vi "Kaelus PIM Add Model with Serial Numbers to Tree.vi"(4 "Instrument Index":i32, 6 "Model Serial Numbers":string[](array[string]), 8 "error in (no error)":errorcluster, 9 "Model Descriptive Columns":string[](array[string]), 10 "Model Name":string="Model", 11 "Tree Control Reference":refnum<vi>) -> (0 "error out":errorcluster)   [LabVIEW 2011]
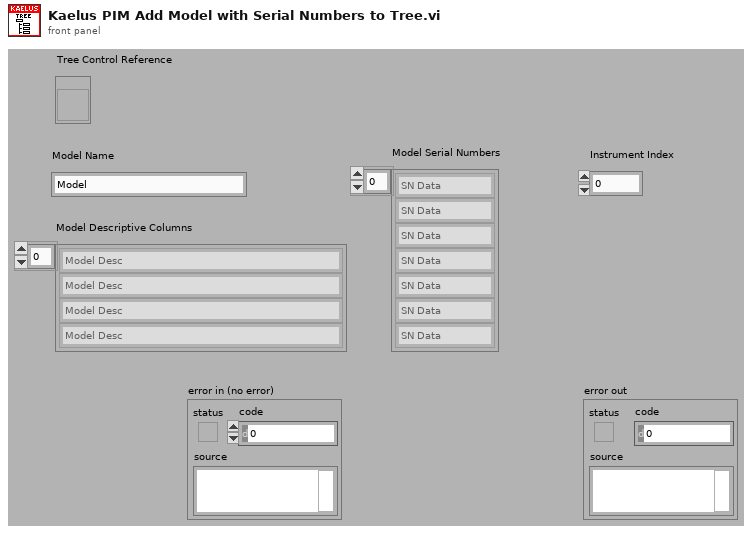
[diagram p1: front panel]
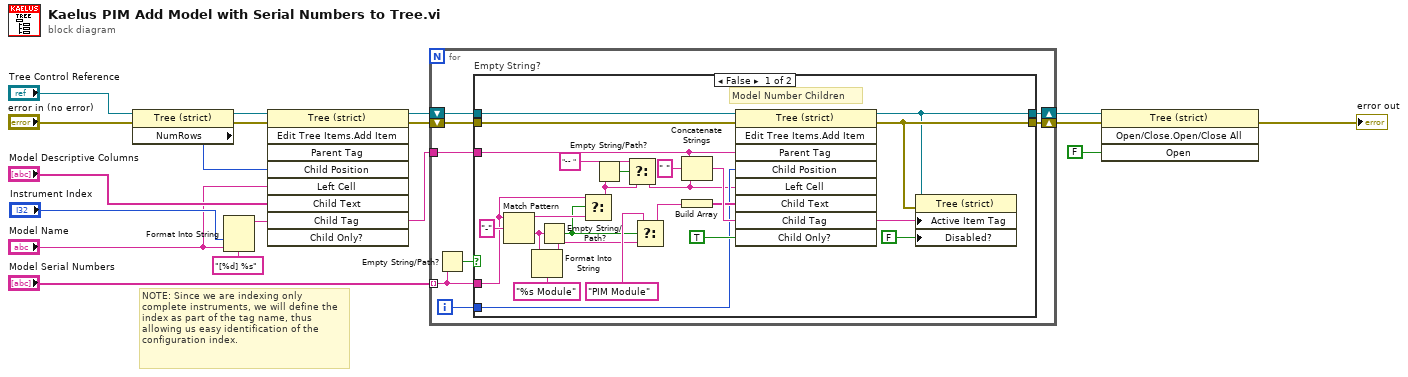
[diagram p0: block diagram]
diagram:
  # "NOTE: Since we are indexing only complete instruments, we will define the index as part of the tag name, thus allowing us easy identification of the configuration index."
  n1 = property class="Tree (strict)"(reference="Tree Control Reference", error in="error in (no error)") -> (reference out=w3:refnum<vi>, error out=w2:errorcluster, "NumRows"=w1:u32)
  n2 = Format Into String(format string="[%d] %s", "Instrument Index", "Model Name") -> (resulting string=w17:string)  [unwired: 2 in, 1 out]
  n3 = invoke class="Tree (strict)" method="Edit Tree Items.Add Item"(reference=w3, error in=w2, "Child Position"=w1, "Left Cell"="Model Name", "Child Text"="Model Descriptive Columns", "Child Tag"=w17) -> (reference out=w16:refnum<vi>, error out=w13:errorcluster)  [unwired: 3 in, 7 out]
  n4 = for {
    tunnel: w17 -> [w21]
    tunnel: "Model Serial Numbers" -> [w18] mode=indexing
    shift-right: [w23] -> w7
    shift-left: w13 -> [w24]
    shift-right: [w22] -> w8
    shift-left: w16 -> [w25]
    i -> [w20]
    n5 = Empty String/Path?(string/path=w18) -> (empty?=w19:bool)
    n6 = case "Empty String?" shown="False" w19 {
      tunnel: w25 -> [w32 w51]
      tunnel: w24 -> [w33 w50]
      tunnel: [w27 w50] -> w23
      tunnel: [w26 w51] -> w22
      tunnel: w18 -> [w37 _]
      tunnel: w21 -> [w36 _]
      tunnel: w20 -> [w34 _]
      frame False {
        # "Model Number Children"
        n7 = Match Pattern(string=w37, regular expression="-") -> (before substring=w39:string, after substring=w43:string)  [unwired: 1 in, 2 out]
        n8 = Format Into String(format string="%s Module", w43) -> (resulting string=w42:string)  [unwired: 2 in, 1 out]
        n9 = Empty String/Path?(string/path=w43) -> (empty?=w38:bool)
        n10 = Select(t=w37, s=w38, f=w39) -> (s? t:f=w30:string)
        n11 = Empty String/Path?(string/path=w30) -> (empty?=w31:bool)
        n12 = Select(t="-- " ("string"), s=w31, f=w30) -> (s? t:f=w29:string)
        n13 = Select(t="PIM Module" ("regular expression"), s=w38, f=w42) -> (s? t:f=w41:string)
        n14 = Concatenate Strings(w36, " " ("string"), w29) -> (w48:string)
        n15 = Build Array(w41) -> (w40:string[])
        n16 = invoke class="Tree (strict)" method="Edit Tree Items.Add Item"(reference=w32, error in=w33, "Parent Tag"=w36, "Child Position"=w34, "Left Cell"=w29, "Child Text"=w40, "Child Tag"=w48, "Child Only?"=TRUE) -> (reference out=w26:refnum<vi>, error out=w27:errorcluster)  [unwired: 1 in, 7 out]
        n17 = property class="Tree (strict)"(reference=w26, error in=w27, "Active Item Tag"=w48, "Disabled?"=FALSE ("Active Item:Disabled?")) -> ()  [unwired: 2 out]
      }
      frame True {
        # "If we receive an empty SN string, don't add it to the tree"
      }
    }
  }
  n18 = invoke class="Tree (strict)" method="Open/Close.Open/Close All"(reference=w8, error in=w7, "Open"=FALSE ("Open?")) -> (error out=→"error out":errorcluster)  [unwired: 1 in, 3 out]
